vi "Rotate Radians.vi"(0 "Radians to Turn":dbl format="%#_13g", 11 "error in":errorcluster) -> (15 "error out":errorcluster)   [LabVIEW 2016]
uses:
  Refname/Motors.ctl
  Refname/Refname to String (Motors).vi
  <vilib>/addons/control/pid/pid.llb/PID (DBL).vi
  <vilib>/addons/control/pid/NI_PID_pid.lvlib
panel:
  in  "Threshold Wheel":dbl format="%#_13g"
  in  "PID Gains Wheel":T1={"proportional gain (Kc)"=1.0, "integral time (Ti, min)"=0.01, "derivative time (Td, min)"=0.0} {"derivative time (Td, min)" format="%.3f"; "integral time (Ti, min)" format="%.3f"; "proportional gain (Kc)" format="%.3f"}
  in  "Threshhold Swerve":dbl
  in  "PID gains Swerve":T1={"proportional gain (Kc)"=1.0, "integral time (Ti, min)"=0.01, "derivative time (Td, min)"=0.0} {"derivative time (Td, min)" format="%.3f"; "integral time (Ti, min)" format="%.3f"; "proportional gain (Kc)" format="%.3f"}
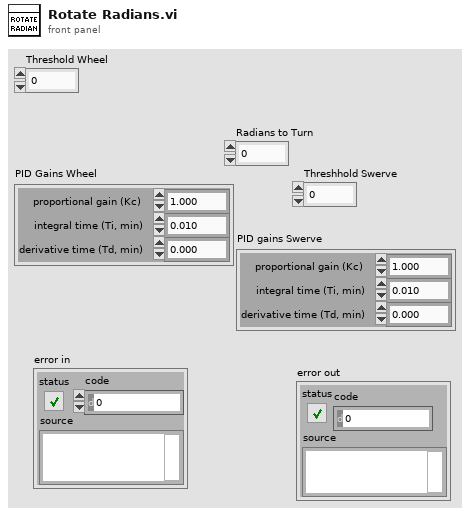
[diagram p1: front panel]
types:
  T1 = cluster{"proportional gain (Kc)":dbl, "integral time (Ti, min)":dbl, "derivative time (Td, min)":dbl}
  T2 = typedef "Motors.ctl" = enum16{"Wheel 1", "Swerve 1", "Wheel 2", "Swerve 2", "Wheel 3", "Swerve 3", "Wheel 4", "Swerve 4"}
  T3 = typedef "WPI_MotorControlDeviceRef.ctl" = cluster{"DeviceStatus":errorcluster, "Type":T4, "PWM":cluster{"PWM Channel":T5, "DeadBand":T6}, "CAN":cluster{"Device Number":u8, "SetOutput VI Ref":variant, "GetOutput VI Ref":variant, "Enable VI Ref":variant, "Disable VI Ref":variant, "Data":variant}, "Invert":bool}
  T4 = typedef "WPI_MotorControlType.ctl" = enum16{"PWM", "CAN"}
  T5 = typedef "FPGA_DIOPWMChannel.ctl" = enum8{"PWM 0", "PWM 1", "PWM 2", "PWM 3", "PWM 4", "PWM 5", "PWM 6", "PWM 7", "PWM 8", "PWM 9", "PWM MXP 0", "PWM MXP 1", "PWM MXP 2", "PWM MXP 3", "PWM MXP 4", "PWM MXP 5", "PWM MXP 6", "PWM MXP 7", "PWM MXP 8", "PWM MXP 9", "Invalid"}
  T6 = typedef "WPI_PWMDeadband.ctl" = cluster{"Name":string, "maxPositivePwm":i32, "minPositivePwm":i32, "centerPwm":i32, "maxNegativePwm":i32, "minNegativePwm":i32, "angularRange":u16}
  T7 = typedef "WPI_CANTalonSRX_GlobalStatus.ctl" = cluster{"Applied Throttle":dbl, "Module Enabled":bool, "CAN Error":errorcluster, "Closed Loop Error":dbl, "Forward Limit Switch Closed":bool, "Reverse Limit Switch Closed":bool, "Sensor Position":dbl, "Sensor Velocity":dbl, "Current":dbl, "Sticky Fault - Over Temp":bool, "Sticky Fault - Under Voltage":bool, "Sticky Fault - Forward Limit":bool, "Sticky Fault - Reverse Limit":bool, "Sticky Fault - Forward Soft Limit":bool, "Sticky Fault - Reverse Soft Limit":bool, "Brake is Enabled":bool, "Encoder Position":dbl, "Encoder Velocity":dbl, "Encoder Index Count":dbl, "Encoder A Pin State":bool, "Encoder B Pin State":bool, "Encoder Index Pin State":bool, "Analog In":dbl, "Analog In Velocity":dbl, "Temperature (C)":dbl, "Battery Voltage":dbl, "Control 5 Is Supported":bool, "Current Profile Slot Select":dbl, "Pos Div 8":bool, "Vel Div 4":bool, "Pulse Width Position":i32, "Pulse Width Velocity":i32, "Pulse Width Rise To Rise (us)":i32, "Pulse Width Rise To Fall (us)":i32, "Mot Prof Active Is Under Run":bool, "Mot Prof Active Has Under Run":bool, "Mot Prof Active Is Last":bool, "Mot Prof Active Velocity Only":bool, "Mot Prof Active Is Valid":bool, "Mot Prof Buffer Is Full":bool, "Mot Prof Active Profile Slot Select":i32, "Mot Prof NextID":i32, "Mot Prof Count":i32, "Mot Prof Active Velocity":dbl, "Mot Prof Active Position":dbl, "Mot Prof Output Enable":i32}
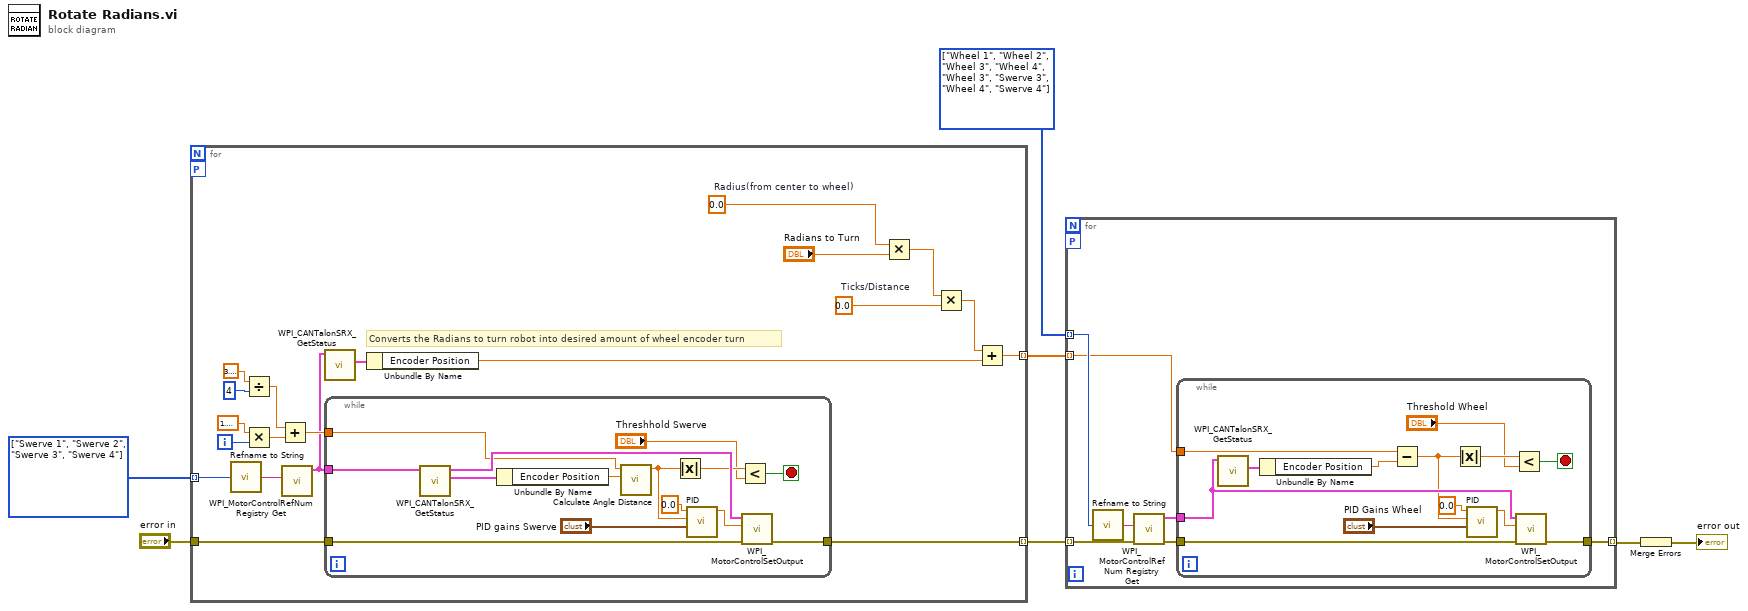
[diagram p0: block diagram]
diagram:
  w6 = T2[] [enum."Swerve 1", enum."Swerve 2", enum."Swerve 3", enum."Swerve 4"] items=["Wheel 1", "Swerve 1", "Wheel 2", "Swerve 2", "Wheel 3", "Swerve 3", "Wheel 4", "Swerve 4"]
  w7 = T2[] [enum."Wheel 1", enum."Wheel 2", enum."Wheel 3", enum."Wheel 4", enum."Wheel 3", enum."Swerve 3", enum."Wheel 4", enum."Swerve 4"] items=["Wheel 1", "Swerve 1", "Wheel 2", "Swerve 2", "Wheel 3", "Swerve 3", "Wheel 4", "Swerve 4"]
  n1 = for {
    workers-P: _ -> [_]
    tunnel: w6 -> [w27] mode=indexing
    tunnel: [w19] -> w5 mode=indexing
    tunnel: [w9] -> w4 mode=indexing
    tunnel: "error in" -> [w8]
    i -> [w26]
    w13 = 0.0  # Ticks/Distance
    w11 = 0.0  # Radius(from center to wheel)
    # "Converts the Radians to turn robot into desired amount of wheel encoder turn"
    n2 = call-poly "Refname to String.vi"("Enum"=w27) -> ("String"=w20:string)
    n3 = Divide(x=3.141592653589793, y=4) -> (x/y=w23:dbl)
    n4 = Multiply(x=1.5707963267948966, y=w26) -> (x*y=w24:dbl)
    n5 = Add(x=w23, y=w24) -> (x+y=w18:dbl)
    n6 = call <vilib>:"WPI_MotorControlRefNum Registry Get.vi"("refnum name"=w20) -> ("MotorControlDevRef"=w16:T3)  [unwired: 9 in, 1 out]
    n7 = call <vilib>:"WPI_CANTalonSRX_GetStatus.vi"("CAN Talon SRX Ref"=w16) -> ("Talon SRX Status"=w17:T7)  [unwired: 8 in, 2 out]
    n8 = while {
      tunnel: [w41] -> w19
      tunnel: w16 -> [w36]
      tunnel: w18 -> [w34]
      tunnel: w8 -> [w28]
      stop <- w30 stop-if-true
      n9 = call <vilib>:"WPI_CANTalonSRX_GetStatus.vi"("CAN Talon SRX Ref"=w36) -> ("Talon SRX Status"=w38:T7, "CAN Talon SRX Ref"=w37:T3)  [unwired: 8 in, 1 out]
      n10 = Unbundle By Name(w38) -> ("Encoder Position"=w35:dbl)
      n11 = call "Calculate Angle Distance.vi"("Current Position"=w35, "Desired Position"=w34) -> ("Distance"=w32:dbl)  [unwired: 9 in]
      n12 = Absolute Value(x=w32) -> (abs(x)=w31:dbl)
      n13 = call-poly <vilib>:"PID.vi"("PID gains"="PID gains Swerve", "process variable"=w32, "setpoint"=0.0) -> ("output"=w33:dbl)  [unwired: 7 in, 1 out]
      n14 = Less?(x=w31, y="Threshhold Swerve") -> (x < y?=w30:bool)
      n15 = call <vilib>:"WPI_MotorControlSetOutput.vi"("error in (no error)"=w28, "Output"=w33, "MotorControlDevRef"=w37) -> ("error out"=w41:errorcluster)  [unwired: 6 in, 2 out]
    }
    n16 = Unbundle By Name(w17) -> ("Encoder Position"=w10:dbl)
    n17 = Multiply(x=w11, y="Radians to Turn") -> (x*y=w14:dbl)
    n18 = Multiply(x=w14, y=w13) -> (x*y=w15:dbl)
    n19 = Add(x=w15, y=w10) -> (x+y=w9:dbl)
  }
  n20 = for {
    workers-P: _ -> [_]
    tunnel: w7 -> [w46] mode=indexing
    tunnel: w4 -> [w45] mode=indexing
    tunnel: w5 -> [w43] mode=indexing
    tunnel: [w42] -> w2 mode=indexing
    n21 = call-poly "Refname to String.vi"("Enum"=w46) -> ("String"=w48:string)
    n22 = call <vilib>:"WPI_MotorControlRefNum Registry Get.vi"("error in (no error)"=w43, "refnum name"=w48) -> ("error out"=w47:errorcluster, "MotorControlDevRef"=w44:T3)  [unwired: 8 in]
    n23 = while {
      tunnel: w47 -> [w59]
      tunnel: w45 -> [w57]
      tunnel: w44 -> [w60]
      tunnel: [w49] -> w42
      stop <- w50 stop-if-true
      n24 = call <vilib>:"WPI_CANTalonSRX_GetStatus.vi"("CAN Talon SRX Ref"=w60) -> ("Talon SRX Status"=w61:T7)  [unwired: 8 in, 2 out]
      n25 = Unbundle By Name(w61) -> ("Encoder Position"=w56:dbl)
      n26 = Subtract(x=w57, y=w56) -> (x-y=w51:dbl)
      n27 = Absolute Value(x=w51) -> (abs(x)=w53:dbl)
      n28 = call-poly <vilib>:"PID.vi"("PID gains"="PID Gains Wheel", "process variable"=w51, "setpoint"=0.0) -> ("output"=w54:dbl)  [unwired: 7 in, 1 out]
      n29 = Less?(x=w53, y="Threshold Wheel") -> (x < y?=w50:bool)
      n30 = call <vilib>:"WPI_MotorControlSetOutput.vi"("error in (no error)"=w59, "Output"=w54, "MotorControlDevRef"=w60) -> ("error out"=w49:errorcluster)  [unwired: 6 in, 2 out]
    }
  }
  n31 = Merge Errors(w2) -> (→"error out":errorcluster)
